vi "Display File in Notepad.vi"(8 "error in":errorcluster, 11 "File Path":path) -> (0 "error out":errorcluster)   [LabVIEW 2019]
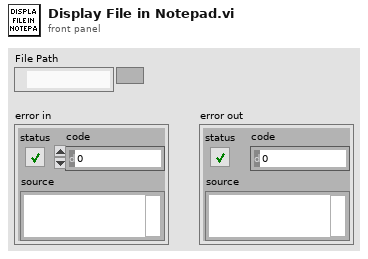
[diagram p1: front panel]
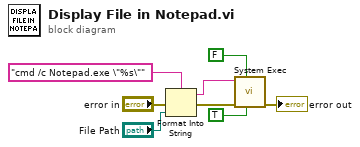
[diagram p0: block diagram]
diagram:
  n1 = Format Into String(format string="cmd /c Notepad.exe \"%s\"" ("command line"), error in="error in", "File Path") -> (resulting string=w1:string, error out=w2:errorcluster)  [unwired: 1 in]
  n2 = call <vilib>:"System Exec.vi"("run minimized? (F)"=TRUE, "wait until completion? (T)"=FALSE, "error in (no error)"=w2, "command line"=w1) -> ("error out"=→"error out":errorcluster)  [unwired: 4 in, 3 out]
